vi "Setup.vi"(7 "ConcreteActor":refnum<class "ConcreteActor.lvclass">) -> (4 "Error":errorcluster, 5 "ConcreteActor":refnum<class "ConcreteActor.lvclass">)   [LabVIEW 2020, in "jettl.lvlib" / "Base.lvlib" / "ConcreteActor.lvclass"]
uses:
  ConcreteActor.lvclass
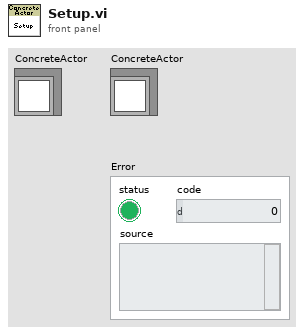
[diagram p1: front panel]
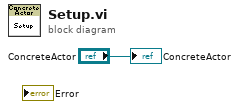
[diagram p0: block diagram]
diagram:
  "ConcreteActor" <- "ConcreteActor"
